vi "Pigeon Gyro.vi"(0 "Reset Yaw?":bool) -> (1 "YPR.Yaw":dbl, 2 "YPR.Yaw Rate":dbl)   [LabVIEW 2017, in "Support Code.lvlib"]
uses:
  Support Code.lvlib
  Public/Documents/Cross The Road Electronics/Phoenix-LabVIEW/Pigeon IMU/CTRE_PigeonIMU_GetYPR.vi
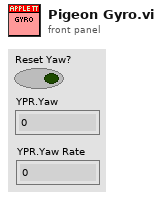
[diagram p1: front panel]
types:
  T1 = typedef "CTRE_PigeonIMU_DeviceRef.ctl" = cluster{"DeviceStatus":errorcluster, "Device Number":u8, "Type":T2, "Device ID":u32, "Handle":u64, "UsageFrame":u32, "Library Path":path}
  T2 = typedef "CTRE_PigeonIMU_ConnectionType.ctl" = u32
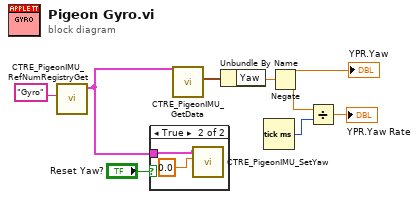
[diagram p0: block diagram]
diagram:
  n1 = call "CTRE_PigeonIMU_RefNumRegistryGet.vi"("refnum name"="Gyro") -> ("PigeonIMUDevRef"=w2:T1)  [unwired: 9 in, 1 out]
  n2 = case shown="True" "Reset Yaw?" {
    tunnel: w2 -> [_ w10]
    frame False {
    }
    frame True {
      n3 = call "CTRE_PigeonIMU_SetYaw.vi"("Value"=0.0, "PigeonIMUDevRef"=w10) -> ()  [unwired: 8 in, 2 out]
    }
  }
  n4 = call-poly "CTRE_PigeonIMU_GetData.vi"("PigeonIMUDevRef"=w2) -> ("Yaw Pitch Roll"=w3:cluster{"Yaw":dbl, "Pitch":dbl, "Roll":dbl})  [unwired: 8 in, 2 out]
  n5 = Unbundle By Name(w3) -> ("Yaw"=w5:dbl)
  n6 = Tick Count (ms)() -> (millisecond timer value=w7:u32)
  n7 = Negate(x=w5) -> (-x=w1:dbl)
  "YPR.Yaw" <- w1
  n8 = Divide(x=w1, y=w7) -> (x/y=→"YPR.Yaw Rate":dbl)
